vi "Get User Info.vi"(2 "错误输入":errorcluster) -> (0 "error out":errorcluster, 1 "UserInfo":string[](array[string]))   [LabVIEW 2013]
panel:
  # "获取登录用户的用户名与密码"
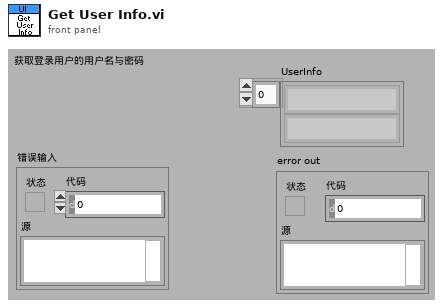
[diagram p1: front panel]
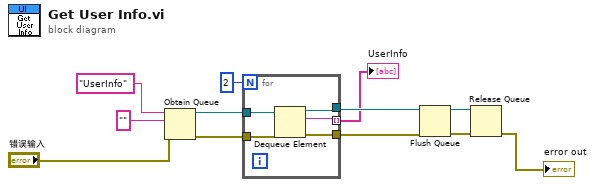
[diagram p0: block diagram]
diagram:
  n1 = Obtain Queue(name (unnamed)="UserInfo" ("名称（未命名）"), element data type="" ("名称（未命名）"), error in (no error)="错误输入") -> (queue out=w4:refnum<queue>, error out=w5:errorcluster)  [unwired: 2 in, 1 out]
  n2 = for {
    N: 2 -> [_]
    tunnel: w4 -> [w17]
    tunnel: w5 -> [w16]
    tunnel: [w15] -> w6 mode=indexing
    tunnel: [w14] -> w7
    tunnel: [w13] -> w8
    n3 = Dequeue Element(queue=w17, error in (no error)=w16) -> (queue out=w14:refnum<queue>, element=w15:string, error out=w13:errorcluster)  [unwired: 1 in, 1 out]
  }
  "UserInfo" <- w6
  n4 = Flush Queue(queue=w7, error in (no error)=w8) -> (queue out=w9:refnum<queue>, error out=w10:errorcluster)  [unwired: 1 out]
  n5 = Release Queue(queue=w9, error in (no error)=w10) -> (error out=→"error out":errorcluster)  [unwired: 1 in, 2 out]
